vi "Global_Variables.vi"() -> ()   [LabVIEW 2019]
panel:
  in  "Press Transducer":u16(ring) items=["500 PSI", "1000 PSI"]
  in  "Cal Channel":dbl[](array[numeric])
  out "Auto Cal":bool
  out "Cancel Add":bool
  in  "Min Max Ring":u16(ring) items=["Minimum", "Maximum"]
  out "Check":bool
  out "Cal complete":bool
  in  "Cal - Minimum":dbl
  in  "Cal - Maximum":dbl
  in  "Cal - b Val":dbl[](array[numeric])
  in  "Cal - x Value":dbl[](array[numeric])
  in  "Cal - Max Val":dbl[](array[numeric])
  in  "Cal - Min Val":dbl[](array[numeric])
  in  "Range String":string[](array[string])
  in  "Type String":string[](array[string])
  in  "Name":string[](array[string])
  out "Calibrate":bool[](array[boolean])
  in  "Range Num":dbl[](array[numeric])
  in  "Type Num":dbl[](array[numeric])
  in  "Channel Num":dbl[](array[numeric])
  in  "Test File Path":path
  in  "COM Port":refnum<visa-resource-name>
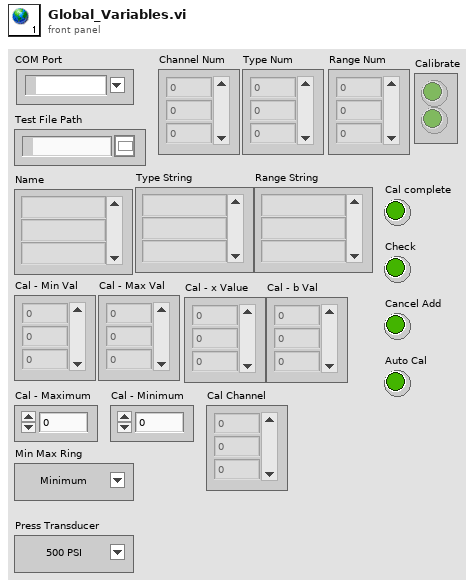
[diagram p1: front panel]
diagram:
